vi "Recognition.Compara.vi"(8 "error in":errorcluster, 9 "SemSenha":bool, 10 "SenhaCadastrada":i32[](array[numeric]), 11 "Senha":string) -> (0 "error out":errorcluster, 3 "SenhaOk":bool)   [LabVIEW 2019]
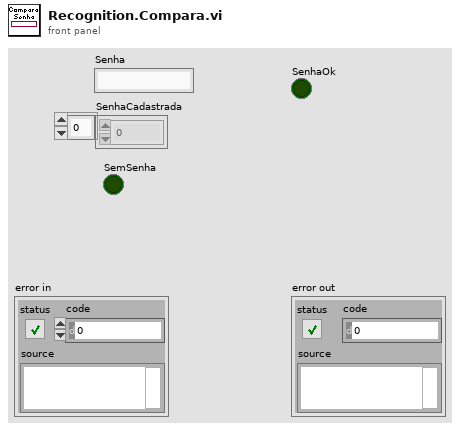
[diagram p1: front panel]
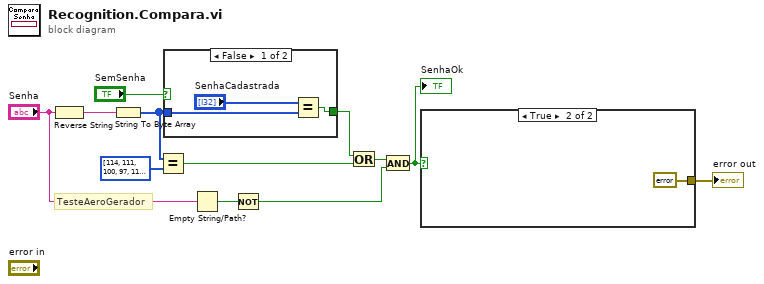
[diagram p0: block diagram]
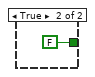
[diagram p2: hidden frame]
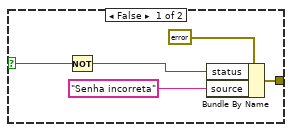
[diagram p3: hidden frame]
diagram:
  # "TesteAeroGerador"
  n1 = Reverse String(1:"Senha") -> (0:w12:string)
  n2 = String To Byte Array(string=w12) -> (unsigned byte array=w7:u8[])
  n3 = Equal?(x=w7, y=u8[] [114, 111, 100, 97, 114, 101, 71, 111, 114, 101, 65, 101, 116, 115, 101, 84] ("unsigned byte array")) -> (x = y?=w9:bool)
  n4 = case shown="False" "SemSenha" {
    tunnel: w7 -> [w15 _]
    tunnel: [w13 FALSE] -> w6
    frame False {
      n5 = Equal?(x="SenhaCadastrada", y=w15) -> (x = y?=w13:bool)
    }
    frame True {
    }
  }
  n6 = Empty String/Path?(string/path="Senha") -> (empty?=w2:bool)
  n7 = Not(x=w2) -> (.not. x?=w1:bool)
  n8 = Or(x=w6, y=w9) -> (x .or. y?=w4:bool)
  n9 = And(x=w4, y=w1) -> (x .and. y?=w3:bool)
  "SenhaOk" <- w3
  n10 = case shown="True" w3 {
    selector: w3 -> [w18 _]
    tunnel: [w20 errorcluster {"status"=FALSE, "code"=0, "source"=""} ("error constant")] -> w11
    frame False {
      n11 = Not(x=w18) -> (.not. x?=w19:bool)
      n12 = Bundle By Name(cluster=errorcluster {"status"=FALSE, "code"=0, "source"=""} ("error constant"), "status"=w19, "source"="Senha incorreta") -> (w20:errorcluster)
    }
    frame True {
    }
  }
  "error out" <- w11
